vi "UI - All UI Objects Refs Memory.vi"(7 "Operation":T1, 8 "error in":errorcluster, 11 "VI Name (\"\" = Caller)":string) -> (0 "error out":errorcluster, 3 "Variant Out":variant)   [LabVIEW 2011]
uses:
  Controls/UI - All UI Objects Refs Memory - Operation.ctl
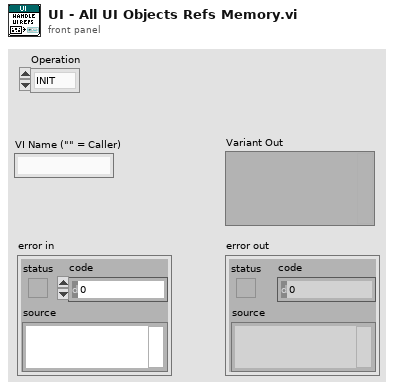
[diagram p1: front panel]
types:
  T1 = typedef "UI - All UI Objects Refs Memory - Operation.ctl" = enum16{"INIT", "GET", "ADD", "CLOSE ALL"}
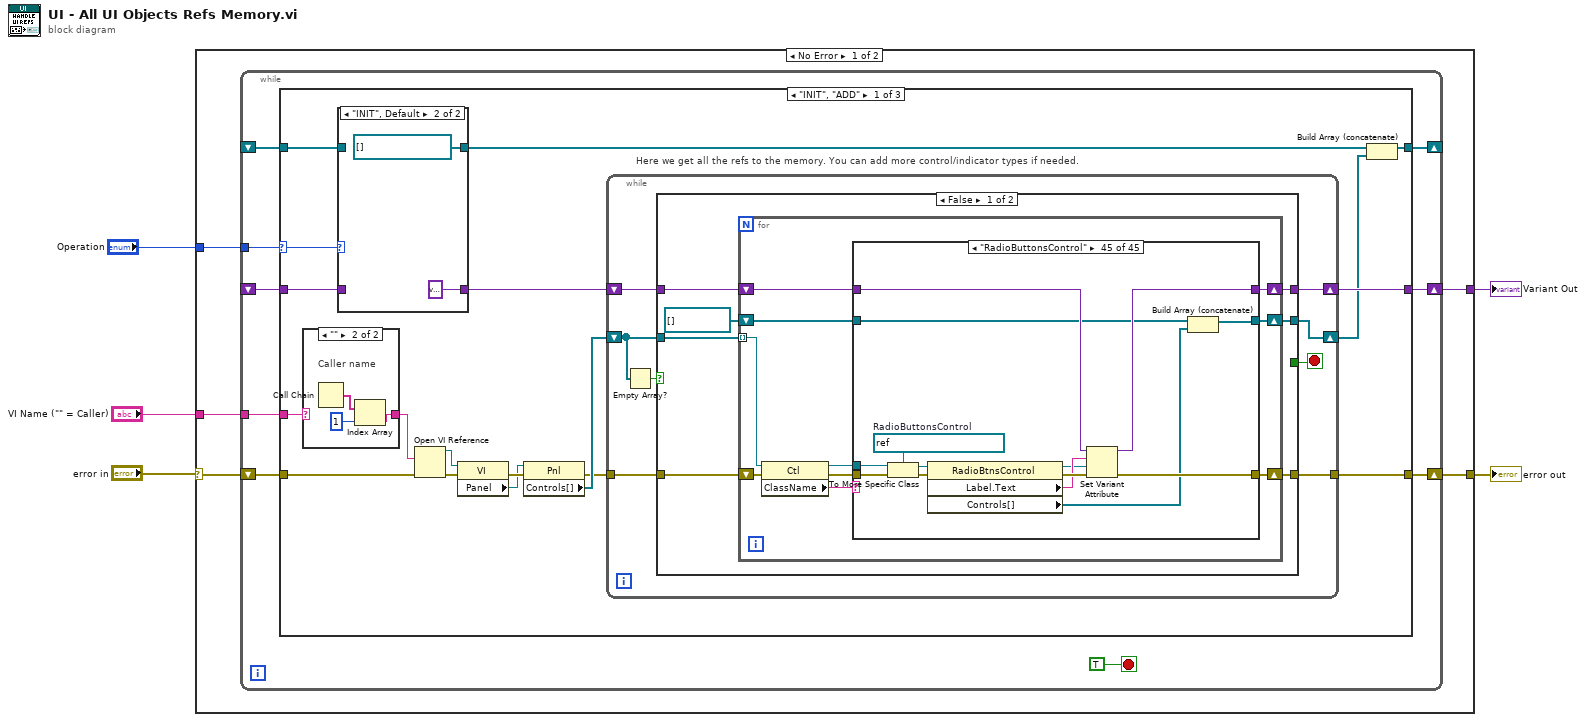
[diagram p0: block diagram]
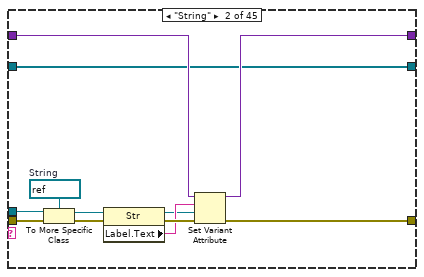
[diagram p3: hidden frame]
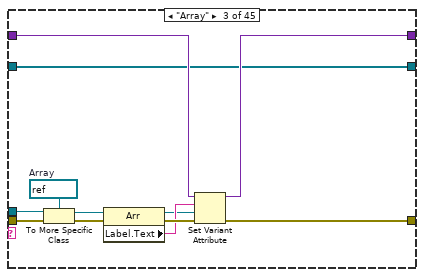
[diagram p4: hidden frame]
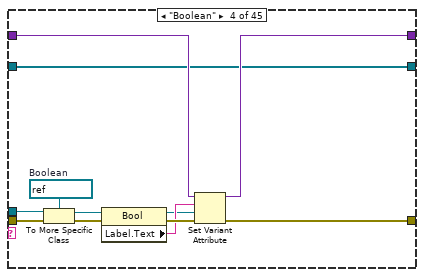
[diagram p5: hidden frame]
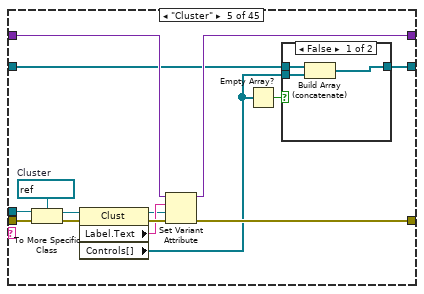
[diagram p6: hidden frame]
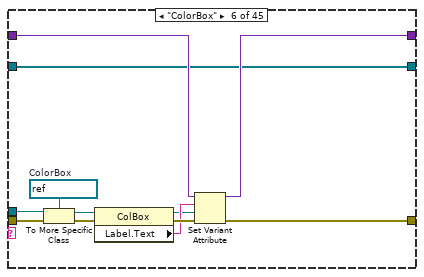
[diagram p8: hidden frame]
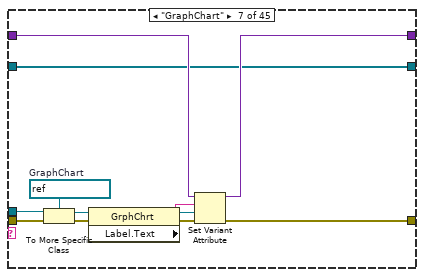
[diagram p9: hidden frame]
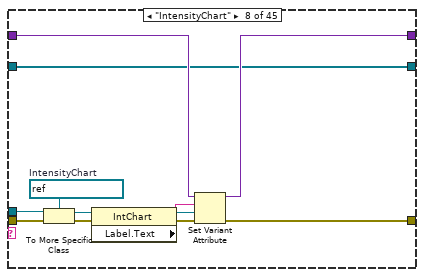
[diagram p10: hidden frame]
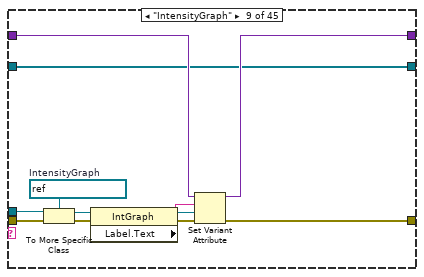
[diagram p11: hidden frame]
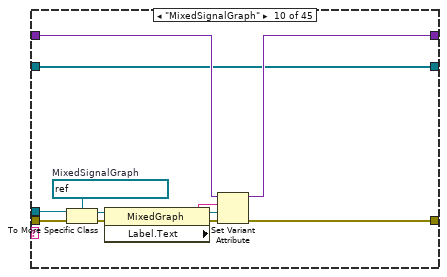
[diagram p12: hidden frame]
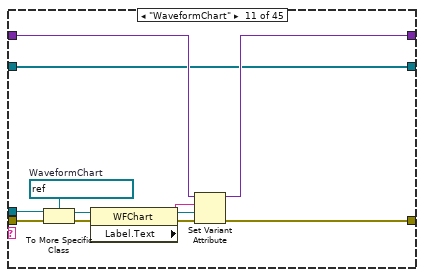
[diagram p13: hidden frame]
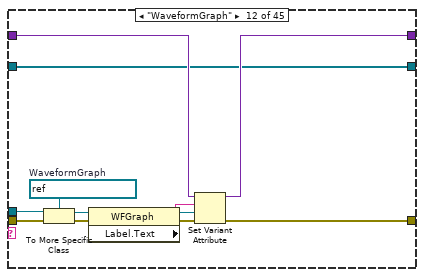
[diagram p14: hidden frame]
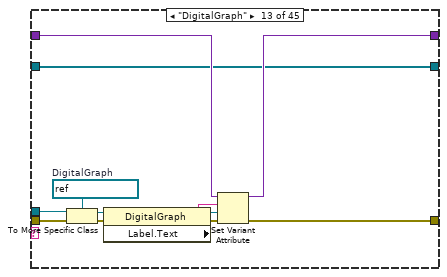
[diagram p15: hidden frame]
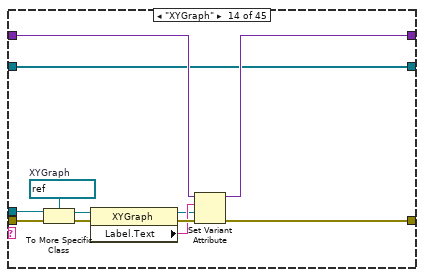
[diagram p16: hidden frame]
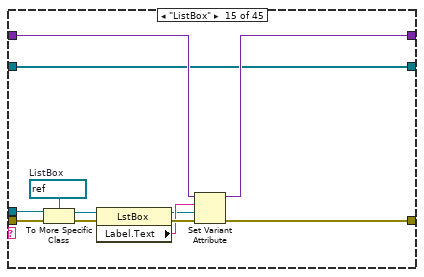
[diagram p17: hidden frame]
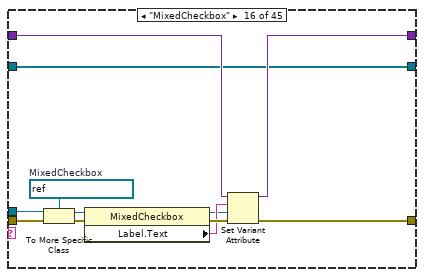
[diagram p18: hidden frame]
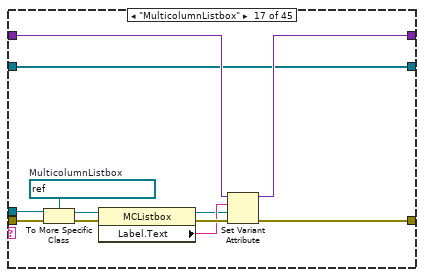
[diagram p19: hidden frame]
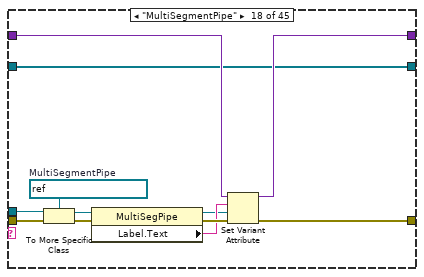
[diagram p20: hidden frame]
diagram:
  n1 = case shown="No Error" "error in" {
    selector: "error in" -> [w9 w629]
    tunnel: [w8 w629] -> w5
    tunnel: "Operation" -> [w10 _]
    tunnel: "VI Name (\"\" = Caller)" -> [w7 _]
    tunnel: [w6 _] -> w1
    frame No Error {
      n2 = while {
        tunnel: w10 -> [w18]
        shift-right: [w13] -> w8
        shift-left: w9 -> [w17]
        tunnel: w7 -> [w16]
        shift-right: [w15] -> w6
        shift-left: _ -> [w14]
        shift-right: [w12] -> _
        shift-left: _ -> [w11]
        stop <- TRUE stop-if-true
        n3 = case shown="\"INIT\", \"ADD\"" w18 {
          selector: w18 -> [w26 _ _]
          tunnel: w17 -> [w37 w625 w628]
          tunnel: w16 -> [w36 _ _]
          tunnel: [w28 _ w627] -> w15
          tunnel: w14 -> [w24 _ w627]
          tunnel: [w27 w624 w628] -> w13
          tunnel: [w22 _ w626] -> w12
          tunnel: w11 -> [w21 w623 w626]
          frame "INIT", "ADD" {
            # "Here we get all the refs to the memory. You can add more control/indicator types if needed."
            n4 = case shown="\"\"" w36 {
              selector: w36 -> [w619 _]
              tunnel: [w619 w620] -> w35
              frame Default {
              }
              frame "" {
                # "Caller name"
                n5 = Call Chain() -> (call chain=w622:string[])
                n6 = Index Array(array=w622, index=1) -> (element=w620:string)
              }
            }
            n7 = case shown="\"INIT\", Default" w26 {
              tunnel: [w616 variant] -> w25
              tunnel: w24 -> [w616 _]
              tunnel: w21 -> [w615 _]
              tunnel: [w615 refnum<vi>[] []] -> w20
              frame "ADD" {
              }
              frame "INIT", Default {
              }
            }
            n8 = Open VI Reference(vi path=w35, error in (no error)=w37) -> (vi reference=w33:refnum<vi>, error out=w34:errorcluster)  [unwired: 4 in]
            n9 = property class="VI"(reference=w33, error in=w34) -> (error out=w32:errorcluster, "Panel"=w31:refnum<vi>)  [unwired: 1 out]
            n10 = property class="Pnl"(reference=w31, error in=w32) -> (error out=w29:errorcluster, "Controls[]"=w30:refnum<vi>[])  [unwired: 1 out]
            n11 = while {
              tunnel: w29 -> [w45]
              tunnel: [w43] -> w27
              shift-right: [w41] -> w23
              shift-left: w30 -> [w40]
              shift-right: [w44] -> w28
              shift-left: w25 -> [w42]
              stop <- w38 stop-if-true
              n12 = Empty Array?(array=w40) -> (empty?=w39:bool)
              n13 = case shown="False" w39 {
                tunnel: w40 -> [w52 _]
                tunnel: w45 -> [w51 w614]
                tunnel: [w50 w613] -> w44
                tunnel: [w49 w614] -> w43
                tunnel: w42 -> [w48 w613]
                tunnel: [w47 _] -> w41
                tunnel: [_ TRUE] -> w38
                frame False {
                  n14 = for {
                    tunnel: w52 -> [w61] mode=indexing
                    shift-right: [w55] -> w49
                    shift-left: w51 -> [w62]
                    shift-right: [w57] -> w50
                    shift-left: w48 -> [w56]
                    shift-right: [w54] -> w47
                    shift-left: refnum<vi>[] [] ("Controls[]") -> [w53]
                    n15 = property class="Ctl"(reference=w61, error in=w62) -> (reference out=w58:refnum<vi>, error out=w60:errorcluster, "ClassName"=w59:string)
                    n16 = case shown="\"RadioButtonsControl\"" w59 {
                      tunnel: w60 -> [w64 w77 w89 w101 w116 w132 w144 w156 w168 w180 w192 w204 w216 w228 w240 w252 w264 w276 w288 w300 w312 w324 w336 w348 w360 w372 w384 w396 w411 w429 w441 w453 w465 w477 w489 w501 w513 w525 w537 w549 w561 w573 w585 w597 w611]
                      tunnel: w58 -> [_ w76 w88 w100 w115 w131 w143 w155 w167 w179 w191 w203 w215 w227 w239 w251 w263 w275 w287 w299 w311 w323 w335 w347 w359 w371 w383 w395 w410 w428 w440 w452 w464 w476 w488 w500 w512 w524 w536 w548 w560 w572 w584 w596 w610]
                      tunnel: [w65 w71 w83 w95 w110 w126 w138 w150 w162 w174 w186 w198 w210 w222 w234 w246 w258 w270 w282 w294 w306 w318 w330 w342 w354 w366 w378 w390 w405 w423 w435 w447 w459 w471 w483 w495 w507 w519 w531 w543 w555 w567 w579 w591 w605] -> w57
                      tunnel: w56 -> [w65 w70 w82 w94 w109 w125 w137 w149 w161 w173 w185 w197 w209 w221 w233 w245 w257 w269 w281 w293 w305 w317 w329 w341 w353 w365 w377 w389 w404 w422 w434 w446 w458 w470 w482 w494 w506 w518 w530 w542 w554 w566 w578 w590 w604]
                      tunnel: [w64 w67 w79 w91 w106 w122 w134 w146 w158 w170 w182 w194 w206 w218 w230 w242 w254 w266 w278 w290 w302 w314 w326 w338 w350 w362 w374 w386 w399 w419 w431 w443 w455 w467 w479 w491 w503 w515 w527 w539 w551 w563 w575 w587 w601] -> w55
                      tunnel: [w63 w66 w78 w90 w105 w121 w133 w145 w157 w169 w181 w193 w205 w217 w229 w241 w253 w265 w277 w289 w301 w313 w325 w337 w349 w361 w373 w385 w397 w418 w430 w442 w454 w466 w478 w490 w502 w514 w526 w538 w550 w562 w574 w586 w598] -> w54
                      tunnel: w53 -> [w63 w66 w78 w90 w104 w121 w133 w145 w157 w169 w181 w193 w205 w217 w229 w241 w253 w265 w277 w289 w301 w313 w325 w337 w349 w361 w373 w385 w398 w418 w430 w442 w454 w466 w478 w490 w502 w514 w526 w538 w550 w562 w574 w586 w599]
                      frame Default {
                        # "Not implemented"
                      }
                      frame "String" {
                        w73 = refnum<vi> refnum  # String
                        n17 = To More Specific Class(target class=w73, reference=w76, error in=w77) -> (specific class reference=w75:refnum<vi>, error out=w74:errorcluster)
                        n18 = property class="Str"(reference=w75, error in=w74) -> (reference out=w68:refnum<vi>, error out=w72:errorcluster, "Label.Text"=w69:string)
                        n19 = Set Variant Attribute(Variant=w70, name=w69, value=w68, error in=w72) -> (Variant out=w71:variant, error out=w67:errorcluster)  [unwired: 1 out]
                      }
                      frame "Array" {
                        w85 = refnum<vi> refnum  # Array
                        n20 = To More Specific Class(target class=w85, reference=w88, error in=w89) -> (specific class reference=w87:refnum<vi>, error out=w86:errorcluster)
                        n21 = property class="Arr"(reference=w87, error in=w86) -> (reference out=w80:refnum<vi>, error out=w84:errorcluster, "Label.Text"=w81:string)
                        n22 = Set Variant Attribute(Variant=w82, name=w81, value=w80, error in=w84) -> (Variant out=w83:variant, error out=w79:errorcluster)  [unwired: 1 out]
                      }
                      frame "Boolean" {
                        w97 = refnum<vi> refnum  # Boolean
                        n23 = To More Specific Class(target class=w97, reference=w100, error in=w101) -> (specific class reference=w99:refnum<vi>, error out=w98:errorcluster)
                        n24 = property class="Bool"(reference=w99, error in=w98) -> (reference out=w92:refnum<vi>, error out=w96:errorcluster, "Label.Text"=w93:string)
                        n25 = Set Variant Attribute(Variant=w94, name=w93, value=w92, error in=w96) -> (Variant out=w95:variant, error out=w91:errorcluster)  [unwired: 1 out]
                      }
                      frame "Cluster" {
                        w112 = refnum<vi> refnum  # Cluster
                        n26 = To More Specific Class(target class=w112, reference=w115, error in=w116) -> (specific class reference=w114:refnum<vi>, error out=w113:errorcluster)
                        n27 = property class="Clust"(reference=w114, error in=w113) -> (reference out=w107:refnum<vi>, error out=w111:errorcluster, "Label.Text"=w108:string, "Controls[]"=w103:refnum<vi>[])
                        n28 = Set Variant Attribute(Variant=w109, name=w108, value=w107, error in=w111) -> (Variant out=w110:variant, error out=w106:errorcluster)  [unwired: 1 out]
                        n29 = Empty Array?(array=w103) -> (empty?=w102:bool)
                        n30 = case shown="False" w102 {
                          tunnel: w103 -> [w119 _]
                          tunnel: [w118 w120] -> w105
                          tunnel: w104 -> [w117 w120]
                          frame False {
                            n31 = Build Array (concatenate)(w117, w119) -> (w118:refnum<vi>[])
                          }
                          frame True {
                          }
                        }
                      }
                      frame "ColorBox" {
                        w128 = refnum<vi> refnum  # ColorBox
                        n32 = To More Specific Class(target class=w128, reference=w131, error in=w132) -> (specific class reference=w130:refnum<vi>, error out=w129:errorcluster)
                        n33 = property class="ColBox"(reference=w130, error in=w129) -> (reference out=w123:refnum<vi>, error out=w127:errorcluster, "Label.Text"=w124:string)
                        n34 = Set Variant Attribute(Variant=w125, name=w124, value=w123, error in=w127) -> (Variant out=w126:variant, error out=w122:errorcluster)  [unwired: 1 out]
                      }
                      frame "GraphChart" {
                        w140 = refnum<vi> refnum  # GraphChart
                        n35 = To More Specific Class(target class=w140, reference=w143, error in=w144) -> (specific class reference=w142:refnum<vi>, error out=w141:errorcluster)
                        n36 = property class="GrphChrt"(reference=w142, error in=w141) -> (reference out=w135:refnum<vi>, error out=w139:errorcluster, "Label.Text"=w136:string)
                        n37 = Set Variant Attribute(Variant=w137, name=w136, value=w135, error in=w139) -> (Variant out=w138:variant, error out=w134:errorcluster)  [unwired: 1 out]
                      }
                      frame "IntensityChart" {
                        w152 = refnum<vi> refnum  # IntensityChart
                        n38 = To More Specific Class(target class=w152, reference=w155, error in=w156) -> (specific class reference=w154:refnum<vi>, error out=w153:errorcluster)
                        n39 = property class="IntChart"(reference=w154, error in=w153) -> (reference out=w147:refnum<vi>, error out=w151:errorcluster, "Label.Text"=w148:string)
                        n40 = Set Variant Attribute(Variant=w149, name=w148, value=w147, error in=w151) -> (Variant out=w150:variant, error out=w146:errorcluster)  [unwired: 1 out]
                      }
                      frame "IntensityGraph" {
                        w164 = refnum<vi> refnum  # IntensityGraph
                        n41 = To More Specific Class(target class=w164, reference=w167, error in=w168) -> (specific class reference=w166:refnum<vi>, error out=w165:errorcluster)
                        n42 = property class="IntGraph"(reference=w166, error in=w165) -> (reference out=w159:refnum<vi>, error out=w163:errorcluster, "Label.Text"=w160:string)
                        n43 = Set Variant Attribute(Variant=w161, name=w160, value=w159, error in=w163) -> (Variant out=w162:variant, error out=w158:errorcluster)  [unwired: 1 out]
                      }
                      frame "MixedSignalGraph" {
                        w176 = refnum<vi> refnum  # MixedSignalGraph
                        n44 = To More Specific Class(target class=w176, reference=w179, error in=w180) -> (specific class reference=w178:refnum<vi>, error out=w177:errorcluster)
                        n45 = property class="MixedGraph"(reference=w178, error in=w177) -> (reference out=w171:refnum<vi>, error out=w175:errorcluster, "Label.Text"=w172:string)
                        n46 = Set Variant Attribute(Variant=w173, name=w172, value=w171, error in=w175) -> (Variant out=w174:variant, error out=w170:errorcluster)  [unwired: 1 out]
                      }
                      frame "WaveformChart" {
                        w188 = refnum<vi> refnum  # WaveformChart
                        n47 = To More Specific Class(target class=w188, reference=w191, error in=w192) -> (specific class reference=w190:refnum<vi>, error out=w189:errorcluster)
                        n48 = property class="WFChart"(reference=w190, error in=w189) -> (reference out=w183:refnum<vi>, error out=w187:errorcluster, "Label.Text"=w184:string)
                        n49 = Set Variant Attribute(Variant=w185, name=w184, value=w183, error in=w187) -> (Variant out=w186:variant, error out=w182:errorcluster)  [unwired: 1 out]
                      }
                      frame "WaveformGraph" {
                        w200 = refnum<vi> refnum  # WaveformGraph
                        n50 = To More Specific Class(target class=w200, reference=w203, error in=w204) -> (specific class reference=w202:refnum<vi>, error out=w201:errorcluster)
                        n51 = property class="WFGraph"(reference=w202, error in=w201) -> (reference out=w195:refnum<vi>, error out=w199:errorcluster, "Label.Text"=w196:string)
                        n52 = Set Variant Attribute(Variant=w197, name=w196, value=w195, error in=w199) -> (Variant out=w198:variant, error out=w194:errorcluster)  [unwired: 1 out]
                      }
                      frame "DigitalGraph" {
                        w212 = refnum<vi> refnum  # DigitalGraph
                        n53 = To More Specific Class(target class=w212, reference=w215, error in=w216) -> (specific class reference=w214:refnum<vi>, error out=w213:errorcluster)
                        n54 = property class="DigitalGraph"(reference=w214, error in=w213) -> (reference out=w207:refnum<vi>, error out=w211:errorcluster, "Label.Text"=w208:string)
                        n55 = Set Variant Attribute(Variant=w209, name=w208, value=w207, error in=w211) -> (Variant out=w210:variant, error out=w206:errorcluster)  [unwired: 1 out]
                      }
                      frame "XYGraph" {
                        w224 = refnum<vi> refnum  # XYGraph
                        n56 = To More Specific Class(target class=w224, reference=w227, error in=w228) -> (specific class reference=w226:refnum<vi>, error out=w225:errorcluster)
                        n57 = property class="XYGraph"(reference=w226, error in=w225) -> (reference out=w219:refnum<vi>, error out=w223:errorcluster, "Label.Text"=w220:string)
                        n58 = Set Variant Attribute(Variant=w221, name=w220, value=w219, error in=w223) -> (Variant out=w222:variant, error out=w218:errorcluster)  [unwired: 1 out]
                      }
                      frame "ListBox" {
                        w236 = refnum<vi> refnum  # ListBox
                        n59 = To More Specific Class(target class=w236, reference=w239, error in=w240) -> (specific class reference=w238:refnum<vi>, error out=w237:errorcluster)
                        n60 = property class="LstBox"(reference=w238, error in=w237) -> (reference out=w231:refnum<vi>, error out=w235:errorcluster, "Label.Text"=w232:string)
                        n61 = Set Variant Attribute(Variant=w233, name=w232, value=w231, error in=w235) -> (Variant out=w234:variant, error out=w230:errorcluster)  [unwired: 1 out]
                      }
                      frame "MixedCheckbox" {
                        w248 = refnum<vi> refnum  # MixedCheckbox
                        n62 = To More Specific Class(target class=w248, reference=w251, error in=w252) -> (specific class reference=w250:refnum<vi>, error out=w249:errorcluster)
                        n63 = property class="MixedCheckbox"(reference=w250, error in=w249) -> (reference out=w243:refnum<vi>, error out=w247:errorcluster, "Label.Text"=w244:string)
                        n64 = Set Variant Attribute(Variant=w245, name=w244, value=w243, error in=w247) -> (Variant out=w246:variant, error out=w242:errorcluster)  [unwired: 1 out]
                      }
                      frame "MulticolumnListbox" {
                        w260 = refnum<vi> refnum  # MulticolumnListbox
                        n65 = To More Specific Class(target class=w260, reference=w263, error in=w264) -> (specific class reference=w262:refnum<vi>, error out=w261:errorcluster)
                        n66 = property class="MCListbox"(reference=w262, error in=w261) -> (reference out=w255:refnum<vi>, error out=w259:errorcluster, "Label.Text"=w256:string)
                        n67 = Set Variant Attribute(Variant=w257, name=w256, value=w255, error in=w259) -> (Variant out=w258:variant, error out=w254:errorcluster)  [unwired: 1 out]
                      }
                      frame "MultiSegmentPipe" {
                        w272 = refnum<vi> refnum  # MultiSegmentPipe
                        n68 = To More Specific Class(target class=w272, reference=w275, error in=w276) -> (specific class reference=w274:refnum<vi>, error out=w273:errorcluster)
                        n69 = property class="MultiSegPipe"(reference=w274, error in=w273) -> (reference out=w267:refnum<vi>, error out=w271:errorcluster, "Label.Text"=w268:string)
                        n70 = Set Variant Attribute(Variant=w269, name=w268, value=w267, error in=w271) -> (Variant out=w270:variant, error out=w266:errorcluster)  [unwired: 1 out]
                      }
                      frame "Numeric" {
                        w284 = refnum<vi> refnum  # Numeric
                        n71 = To More Specific Class(target class=w284, reference=w287, error in=w288) -> (specific class reference=w286:refnum<vi>, error out=w285:errorcluster)
                        n72 = property class="Num"(reference=w286, error in=w285) -> (reference out=w279:refnum<vi>, error out=w283:errorcluster, "Label.Text"=w280:string)
                        n73 = Set Variant Attribute(Variant=w281, name=w280, value=w279, error in=w283) -> (Variant out=w282:variant, error out=w278:errorcluster)  [unwired: 1 out]
                      }
                      frame "ColorRamp" {
                        w296 = refnum<vi> refnum  # ColorRamp
                        n74 = To More Specific Class(target class=w296, reference=w299, error in=w300) -> (specific class reference=w298:refnum<vi>, error out=w297:errorcluster)
                        n75 = property class="ColRmp"(reference=w298, error in=w297) -> (reference out=w291:refnum<vi>, error out=w295:errorcluster, "Label.Text"=w292:string)
                        n76 = Set Variant Attribute(Variant=w293, name=w292, value=w291, error in=w295) -> (Variant out=w294:variant, error out=w290:errorcluster)  [unwired: 1 out]
                      }
                      frame "Digital" {
                        w308 = refnum<vi> refnum  # Digital
                        n77 = To More Specific Class(target class=w308, reference=w311, error in=w312) -> (specific class reference=w310:refnum<vi>, error out=w309:errorcluster)
                        n78 = property class="DigNum"(reference=w310, error in=w309) -> (reference out=w303:refnum<vi>, error out=w307:errorcluster, "Label.Text"=w304:string)
                        n79 = Set Variant Attribute(Variant=w305, name=w304, value=w303, error in=w307) -> (Variant out=w306:variant, error out=w302:errorcluster)  [unwired: 1 out]
                      }
                      frame "NamedNumeric" {
                        w320 = refnum<vi> refnum  # NamedNumeric
                        n80 = To More Specific Class(target class=w320, reference=w323, error in=w324) -> (specific class reference=w322:refnum<vi>, error out=w321:errorcluster)
                        n81 = property class="NmdNum"(reference=w322, error in=w321) -> (reference out=w315:refnum<vi>, error out=w319:errorcluster, "Label.Text"=w316:string)
                        n82 = Set Variant Attribute(Variant=w317, name=w316, value=w315, error in=w319) -> (Variant out=w318:variant, error out=w314:errorcluster)  [unwired: 1 out]
                      }
                      frame "Enum" {
                        w332 = refnum<vi> refnum  # Enum
                        n83 = To More Specific Class(target class=w332, reference=w335, error in=w336) -> (specific class reference=w334:refnum<vi>, error out=w333:errorcluster)
                        n84 = property class="Enum"(reference=w334, error in=w333) -> (reference out=w327:refnum<vi>, error out=w331:errorcluster, "Label.Text"=w328:string)
                        n85 = Set Variant Attribute(Variant=w329, name=w328, value=w327, error in=w331) -> (Variant out=w330:variant, error out=w326:errorcluster)  [unwired: 1 out]
                      }
                      frame "Ring" {
                        w344 = refnum<vi> refnum  # Ring
                        n86 = To More Specific Class(target class=w344, reference=w347, error in=w348) -> (specific class reference=w346:refnum<vi>, error out=w345:errorcluster)
                        n87 = property class="Ring"(reference=w346, error in=w345) -> (reference out=w339:refnum<vi>, error out=w343:errorcluster, "Label.Text"=w340:string)
                        n88 = Set Variant Attribute(Variant=w341, name=w340, value=w339, error in=w343) -> (Variant out=w342:variant, error out=w338:errorcluster)  [unwired: 1 out]
                      }
                      frame "NumericWithScale" {
                        w356 = refnum<vi> refnum  # NumericWithScale
                        n89 = To More Specific Class(target class=w356, reference=w359, error in=w360) -> (specific class reference=w358:refnum<vi>, error out=w357:errorcluster)
                        n90 = property class="NumWthScl"(reference=w358, error in=w357) -> (reference out=w351:refnum<vi>, error out=w355:errorcluster, "Label.Text"=w352:string)
                        n91 = Set Variant Attribute(Variant=w353, name=w352, value=w351, error in=w355) -> (Variant out=w354:variant, error out=w350:errorcluster)  [unwired: 1 out]
                      }
                      frame "Knob" {
                        w368 = refnum<vi> refnum  # Knob
                        n92 = To More Specific Class(target class=w368, reference=w371, error in=w372) -> (specific class reference=w370:refnum<vi>, error out=w369:errorcluster)
                        n93 = property class="Knob"(reference=w370, error in=w369) -> (reference out=w363:refnum<vi>, error out=w367:errorcluster, "Label.Text"=w364:string)
                        n94 = Set Variant Attribute(Variant=w365, name=w364, value=w363, error in=w367) -> (Variant out=w366:variant, error out=w362:errorcluster)  [unwired: 1 out]
                      }
                      frame "Slide" {
                        w380 = refnum<vi> refnum  # Slide
                        n95 = To More Specific Class(target class=w380, reference=w383, error in=w384) -> (specific class reference=w382:refnum<vi>, error out=w381:errorcluster)
                        n96 = property class="Slide"(reference=w382, error in=w381) -> (reference out=w375:refnum<vi>, error out=w379:errorcluster, "Label.Text"=w376:string)
                        n97 = Set Variant Attribute(Variant=w377, name=w376, value=w375, error in=w379) -> (Variant out=w378:variant, error out=w374:errorcluster)  [unwired: 1 out]
                      }
                      frame "PageSelector" {
                        w392 = refnum<vi> refnum  # PageSelector
                        n98 = To More Specific Class(target class=w392, reference=w395, error in=w396) -> (specific class reference=w394:refnum<vi>, error out=w393:errorcluster)
                        n99 = property class="PageSel"(reference=w394, error in=w393) -> (reference out=w387:refnum<vi>, error out=w391:errorcluster, "Label.Text"=w388:string)
                        n100 = Set Variant Attribute(Variant=w389, name=w388, value=w387, error in=w391) -> (Variant out=w390:variant, error out=w386:errorcluster)  [unwired: 1 out]
                      }
                      frame "TabControl" {
                        w407 = refnum<vi> refnum  # TabControl
                        n101 = To More Specific Class(target class=w407, reference=w410, error in=w411) -> (specific class reference=w409:refnum<vi>, error out=w408:errorcluster)
                        n102 = property class="TabCtl"(reference=w409, error in=w408) -> (reference out=w402:refnum<vi>, error out=w406:errorcluster, "Label.Text"=w403:string, "Pages"=w400:refnum<vi>[])
                        n103 = Set Variant Attribute(Variant=w404, name=w403, value=w402, error in=w406) -> (Variant out=w405:variant, error out=w401:errorcluster)  [unwired: 1 out]
                        n104 = for {
                          tunnel: w400 -> [w416] mode=indexing
                          shift-right: [w415] -> w399
                          shift-left: w401 -> [w417]
                          shift-right: [w412] -> w397
                          shift-left: w398 -> [w414]
                          n105 = property class="Page"(reference=w416, error in=w417) -> (error out=w415:errorcluster, "ControlsOnPage"=w413:refnum<vi>[])  [unwired: 1 out]
                          n106 = Build Array (concatenate)(w414, w413) -> (w412:refnum<vi>[])
                        }
                      }
                      frame "Path" {
                        w425 = refnum<vi> refnum  # Path
                        n107 = To More Specific Class(target class=w425, reference=w428, error in=w429) -> (specific class reference=w427:refnum<vi>, error out=w426:errorcluster)
                        n108 = property class="Path"(reference=w427, error in=w426) -> (reference out=w420:refnum<vi>, error out=w424:errorcluster, "Label.Text"=w421:string)
                        n109 = Set Variant Attribute(Variant=w422, name=w421, value=w420, error in=w424) -> (Variant out=w423:variant, error out=w419:errorcluster)  [unwired: 1 out]
                      }
                      frame "Picture" {
                        w437 = refnum<vi> refnum  # Picture
                        n110 = To More Specific Class(target class=w437, reference=w440, error in=w441) -> (specific class reference=w439:refnum<vi>, error out=w438:errorcluster)
                        n111 = property class="Pict"(reference=w439, error in=w438) -> (reference out=w432:refnum<vi>, error out=w436:errorcluster, "Label.Text"=w433:string)
                        n112 = Set Variant Attribute(Variant=w434, name=w433, value=w432, error in=w436) -> (Variant out=w435:variant, error out=w431:errorcluster)  [unwired: 1 out]
                      }
                      frame "Pixmap" {
                        w449 = refnum<vi> refnum  # Pixmap
                        n113 = To More Specific Class(target class=w449, reference=w452, error in=w453) -> (specific class reference=w451:refnum<vi>, error out=w450:errorcluster)
                        n114 = property class="Pixmap"(reference=w451, error in=w450) -> (reference out=w444:refnum<vi>, error out=w448:errorcluster, "Label.Text"=w445:string)
                        n115 = Set Variant Attribute(Variant=w446, name=w445, value=w444, error in=w448) -> (Variant out=w447:variant, error out=w443:errorcluster)  [unwired: 1 out]
                      }
                      frame "RefNum" {
                        w461 = refnum<vi> refnum  # RefNum
                        n116 = To More Specific Class(target class=w461, reference=w464, error in=w465) -> (specific class reference=w463:refnum<vi>, error out=w462:errorcluster)
                        n117 = property class="Ref"(reference=w463, error in=w462) -> (reference out=w456:refnum<vi>, error out=w460:errorcluster, "Label.Text"=w457:string)
                        n118 = Set Variant Attribute(Variant=w458, name=w457, value=w456, error in=w460) -> (Variant out=w459:variant, error out=w455:errorcluster)  [unwired: 1 out]
                      }
                      frame "LVObjectRefNum" {
                        w473 = refnum<vi> refnum  # LVObjectRefNum
                        n119 = To More Specific Class(target class=w473, reference=w476, error in=w477) -> (specific class reference=w475:refnum<vi>, error out=w474:errorcluster)
                        n120 = property class="LVObjRef"(reference=w475, error in=w474) -> (reference out=w468:refnum<vi>, error out=w472:errorcluster, "Label.Text"=w469:string)
                        n121 = Set Variant Attribute(Variant=w470, name=w469, value=w468, error in=w472) -> (Variant out=w471:variant, error out=w467:errorcluster)  [unwired: 1 out]
                      }
                      frame "VIRefNum" {
                        w485 = refnum<vi> refnum  # VIRefNum
                        n122 = To More Specific Class(target class=w485, reference=w488, error in=w489) -> (specific class reference=w487:refnum<vi>, error out=w486:errorcluster)
                        n123 = property class="VIRef"(reference=w487, error in=w486) -> (reference out=w480:refnum<vi>, error out=w484:errorcluster, "Label.Text"=w481:string)
                        n124 = Set Variant Attribute(Variant=w482, name=w481, value=w480, error in=w484) -> (Variant out=w483:variant, error out=w479:errorcluster)  [unwired: 1 out]
                      }
                      frame "TypedRefNum" {
                        w497 = refnum<vi> refnum  # TypedRefNum
                        n125 = To More Specific Class(target class=w497, reference=w500, error in=w501) -> (specific class reference=w499:refnum<vi>, error out=w498:errorcluster)
                        n126 = property class="TypRef"(reference=w499, error in=w498) -> (reference out=w492:refnum<vi>, error out=w496:errorcluster, "Label.Text"=w493:string)
                        n127 = Set Variant Attribute(Variant=w494, name=w493, value=w492, error in=w496) -> (Variant out=w495:variant, error out=w491:errorcluster)  [unwired: 1 out]
                      }
                      frame "DataValRefNum" {
                        w509 = refnum<vi> refnum  # DataValRefNum
                        n128 = To More Specific Class(target class=w509, reference=w512, error in=w513) -> (specific class reference=w511:refnum<vi>, error out=w510:errorcluster)
                        n129 = property class="DataValRefNum"(reference=w511, error in=w510) -> (reference out=w504:refnum<vi>, error out=w508:errorcluster, "Label.Text"=w505:string)
                        n130 = Set Variant Attribute(Variant=w506, name=w505, value=w504, error in=w508) -> (Variant out=w507:variant, error out=w503:errorcluster)  [unwired: 1 out]
                      }
                      frame "SceneGraphDisplay" {
                        w521 = refnum<vi> refnum  # SceneGraphDisplay
                        n131 = To More Specific Class(target class=w521, reference=w524, error in=w525) -> (specific class reference=w523:refnum<vi>, error out=w522:errorcluster)
                        n132 = property class="SceneGraphDisp"(reference=w523, error in=w522) -> (reference out=w516:refnum<vi>, error out=w520:errorcluster, "Label.Text"=w517:string)
                        n133 = Set Variant Attribute(Variant=w518, name=w517, value=w516, error in=w520) -> (Variant out=w519:variant, error out=w515:errorcluster)  [unwired: 1 out]
                      }
                      frame "Scrollbar" {
                        w533 = refnum<vi> refnum  # Scrollbar
                        n134 = To More Specific Class(target class=w533, reference=w536, error in=w537) -> (specific class reference=w535:refnum<vi>, error out=w534:errorcluster)
                        n135 = property class="Scroll"(reference=w535, error in=w534) -> (reference out=w528:refnum<vi>, error out=w532:errorcluster, "Label.Text"=w529:string)
                        n136 = Set Variant Attribute(Variant=w530, name=w529, value=w528, error in=w532) -> (Variant out=w531:variant, error out=w527:errorcluster)  [unwired: 1 out]
                      }
                      frame "ComboBox" {
                        w545 = refnum<vi> refnum  # ComboBox
                        n137 = To More Specific Class(target class=w545, reference=w548, error in=w549) -> (specific class reference=w547:refnum<vi>, error out=w546:errorcluster)
                        n138 = property class="CmbBox"(reference=w547, error in=w546) -> (reference out=w540:refnum<vi>, error out=w544:errorcluster, "Label.Text"=w541:string)
                        n139 = Set Variant Attribute(Variant=w542, name=w541, value=w540, error in=w544) -> (Variant out=w543:variant, error out=w539:errorcluster)  [unwired: 1 out]
                      }
                      frame "SubPanel" {
                        w557 = refnum<vi> refnum  # SubPanel
                        n140 = To More Specific Class(target class=w557, reference=w560, error in=w561) -> (specific class reference=w559:refnum<vi>, error out=w558:errorcluster)
                        n141 = property class="SubPnl" props=["Label", "Text", "DiagramInserted"](reference=w559, error in=w558) -> (reference out=w552:refnum<vi>, error out=w556:errorcluster, "Label.Text"=w553:string)  [unwired: 1 out]
                        n142 = Set Variant Attribute(Variant=w554, name=w553, value=w552, error in=w556) -> (Variant out=w555:variant, error out=w551:errorcluster)  [unwired: 1 out]
                      }
                      frame "Table" {
                        w569 = refnum<vi> refnum  # Table
                        n143 = To More Specific Class(target class=w569, reference=w572, error in=w573) -> (specific class reference=w571:refnum<vi>, error out=w570:errorcluster)
                        n144 = property class="Tbl"(reference=w571, error in=w570) -> (reference out=w564:refnum<vi>, error out=w568:errorcluster, "Label.Text"=w565:string)
                        n145 = Set Variant Attribute(Variant=w566, name=w565, value=w564, error in=w568) -> (Variant out=w567:variant, error out=w563:errorcluster)  [unwired: 1 out]
                      }
                      frame "TreeControl" {
                        w581 = refnum<vi> refnum  # TreeControl
                        n146 = To More Specific Class(target class=w581, reference=w584, error in=w585) -> (specific class reference=w583:refnum<vi>, error out=w582:errorcluster)
                        n147 = property class="Tree"(reference=w583, error in=w582) -> (reference out=w576:refnum<vi>, error out=w580:errorcluster, "Label.Text"=w577:string)
                        n148 = Set Variant Attribute(Variant=w578, name=w577, value=w576, error in=w580) -> (Variant out=w579:variant, error out=w575:errorcluster)  [unwired: 1 out]
                      }
                      frame "WaveformData" {
                        w593 = refnum<vi> refnum  # WaveformData
                        n149 = To More Specific Class(target class=w593, reference=w596, error in=w597) -> (specific class reference=w595:refnum<vi>, error out=w594:errorcluster)
                        n150 = property class="WFD"(reference=w595, error in=w594) -> (reference out=w588:refnum<vi>, error out=w592:errorcluster, "Label.Text"=w589:string)
                        n151 = Set Variant Attribute(Variant=w590, name=w589, value=w588, error in=w592) -> (Variant out=w591:variant, error out=w587:errorcluster)  [unwired: 1 out]
                      }
                      frame "RadioButtonsControl" {
                        w607 = refnum<vi> refnum  # RadioButtonsControl
                        n152 = To More Specific Class(target class=w607, reference=w610, error in=w611) -> (specific class reference=w609:refnum<vi>, error out=w608:errorcluster)
                        n153 = property class="RadioBtnsControl"(reference=w609, error in=w608) -> (reference out=w602:refnum<vi>, error out=w606:errorcluster, "Label.Text"=w603:string, "Controls[]"=w600:refnum<vi>[])
                        n154 = Set Variant Attribute(Variant=w604, name=w603, value=w602, error in=w606) -> (Variant out=w605:variant, error out=w601:errorcluster)  [unwired: 1 out]
                        n155 = Build Array (concatenate)(w599, w600) -> (w598:refnum<vi>[])
                      }
                    }
                  }
                }
                frame True {
                }
              }
            }
            n156 = Build Array (concatenate)(w20, w23) -> (w22:refnum<vi>[])
          }
          frame "CLOSE ALL" {
            n157 = Close Reference(reference=w623, error in (no error)=w625) -> (error out=w624:errorcluster)
          }
          frame "GET" {
            # "Here we just read out the shift register..."
          }
        }
      }
    }
    frame Error {
    }
  }
  "error out" <- w5
  "Variant Out" <- w1
